vi "facade.vi"(0 "Data In":T13, 2 "Display State In":T3={"current frame index"=0, "number of images"=0, "ROI (frames)"={"ROI"=[]}, "control refs"={"frame"=refnum, "image"=refnum, "saveROIsButton"=refnum, "loadImageSwitch"=refnum, "loadROIsSwitch"=refnum, "saveROIsSwitch"=refnum, "loadImagePath"=refnum, "loadROIPath"=refnum, "redraw"=refnum}, "calibration"={"x"=0.0, "y"=0.0, "x unit"=enum."um", "y unit"=enum."um"}, "xpaths"={"x offset"="", "y offset"="", "z offset"=""}, "offset"=refnum, "XML description"="", "number of ROIs"=0.0, "ROI Tool Buttons Visible"={"Zoom Tool"=FALSE, "Selection Tool"=FALSE, "Pan Tool"=FALSE, "Point Tool"=FALSE, "Line Tool"=FALSE, "Rectangle Tool"=FALSE, "Rotated Rectangle Tool"=FALSE, "Polyline Tool"=FALSE, "Polygon Tool"=FALSE, "Freehand Tool"=FALSE, "Closed Freehand Tool"=FALSE, "Ellipse Tool"=FALSE, "Annulus Tool"=FALSE}, "ROI color"=0, "enable ROI numbering?"=FALSE, "selected path to save ROIs"=path "", "starting path"=path "", "loaded image path"=path "", "array of overlays"=[], "pointCollection"=refnum, "ROImode"=enum."IMAQROIs", "selected point ID"=0.0, "point radius"=0, "point colours"=[], "PlotAreaSize"={"Width"=0, "Height"=0}, "last action"=enum."not specified"} {"array of overlays"."overlay size" min=1}, 3 "Container State":T12, 5 "error in (no error)":errorcluster) -> (4 "error out":errorcluster, 6 "Data Out":T13, 7 "Display State Out":T3={"current frame index"=0, "number of images"=0, "ROI (frames)"={"ROI"=[]}, "control refs"={"frame"=refnum, "image"=refnum, "saveROIsButton"=refnum, "loadImageSwitch"=refnum, "loadROIsSwitch"=refnum, "saveROIsSwitch"=refnum, "loadImagePath"=refnum, "loadROIPath"=refnum, "redraw"=refnum}, "calibration"={"x"=0.0, "y"=0.0, "x unit"=enum."um", "y unit"=enum."um"}, "xpaths"={"x offset"="", "y offset"="", "z offset"=""}, "offset"=refnum, "XML description"="", "number of ROIs"=0.0, "ROI Tool Buttons Visible"={"Zoom Tool"=FALSE, "Selection Tool"=FALSE, "Pan Tool"=FALSE, "Point Tool"=FALSE, "Line Tool"=FALSE, "Rectangle Tool"=FALSE, "Rotated Rectangle Tool"=FALSE, "Polyline Tool"=FALSE, "Polygon Tool"=FALSE, "Freehand Tool"=FALSE, "Closed Freehand Tool"=FALSE, "Ellipse Tool"=FALSE, "Annulus Tool"=FALSE}, "ROI color"=0, "enable ROI numbering?"=FALSE, "selected path to save ROIs"=path "", "starting path"=path "", "loaded image path"=path "", "array of overlays"=[], "pointCollection"=refnum, "ROImode"=enum."IMAQROIs", "selected point ID"=0.0, "point radius"=0, "point colours"=[], "PlotAreaSize"={"Width"=0, "Height"=0}, "last action"=enum."not specified"} {"array of overlays"."overlay size" min=1}, 8 "Action":T2)   [LabVIEW 2010, in "XImage.xctl"]
uses:
  XImage.xctl
  data.ctl
  classes/ImageCollection/ImageCollection/ImageCollection.lvclass
  <vilib>/_xctls/Container State.ctl
  state.ctl
  classes/SpaceVector/SpaceVector/SpaceVector.lvclass
  classes/PointCollection/PointCollection/PointCollection.lvclass
  ROI_frames_cluster.ctl
  control_refs_cluster.ctl
  calibration_cluster.ctl
  enumerations/unit.ctl
  xpath_cluster.ctl
  overlays_cluster.ctl
  ROI_mode_enum.ctl
  last_action_enum.ctl
  <vilib>/_xctls/Action.ctl
  classes/Image/Image/Image.lvclass
  <vilib>/vision/Image Controls.llb/IMAQ Image.ctl
  <vilib>/Utility/inputDevices.llb/keyboardAcquire.vi
  <vilib>/Utility/inputDevices.llb/closeKeyboard.vi
  <vilib>/_xctls/XControlSupport.lvlib
panel:
  in  "button:saveLinear":bool
  out "event case no.":i32
  in  "redraw":bool
  in  "button:savePoints":bool
  in  "button:loadPoints":bool
  in  "showHeaderButton":bool
  in  "loadROIPath":path caption="start path"
  in  "loadImagePath":path
  in  "loadROIsSwitch":bool=TRUE
  in  "saveROIsSwitch":bool=TRUE
  in  "loadImageSwitch":bool=TRUE
  out "progress bar":u8(slide) scale=0.0..100.0
  in  "button:loadROIs":bool
  in  "button:saveROIs":bool
  in  "button:loadImage":bool
  in  "frame":i32(slide) scale=0.0..10.0
  out "Image":T1(plugin-control)
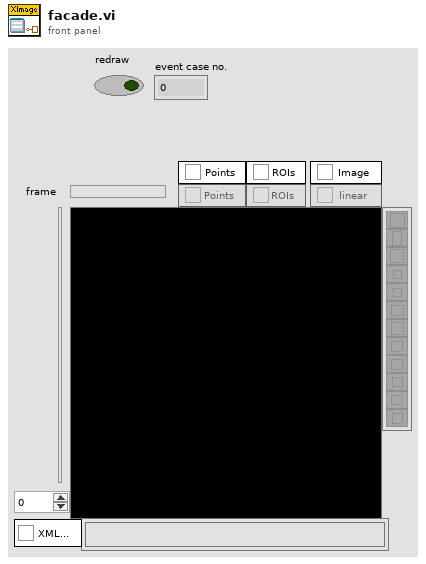
[diagram p1: front panel]
types:
  T1 = typedef "IMAQ Image.ctl" = refnum<image>
  T2 = typedef "XControlSupport.lvlib/Action.ctl" = cluster{"Data Changed?":bool, "State Changed?":bool, "Action Name":string}
  T3 = typedef "XImage.xctl/state.ctl" = cluster{"current frame index":i32, "number of images":i32, "ROI (frames)":T4, "control refs":T5, "calibration":T6, "xpaths":T8, "offset":refnum<class "SpaceVector.lvclass">, "XML description":string, "number of ROIs":dbl, "ROI Tool Buttons Visible":cluster{"Zoom Tool":bool, "Selection Tool":bool, "Pan Tool":bool, "Point Tool":bool, "Line Tool":bool, "Rectangle Tool":bool, "Rotated Rectangle Tool":bool, "Polyline Tool":bool, "Polygon Tool":bool, "Freehand Tool":bool, "Closed Freehand Tool":bool, "Ellipse Tool":bool, "Annulus Tool":bool}, "ROI color":u32, "enable ROI numbering?":bool, "selected path to save ROIs":path, "starting path":path, "loaded image path":path, "array of overlays":T9[], "pointCollection":refnum<class "PointCollection.lvclass">, "ROImode":T10, "selected point ID":dbl, "point radius":i32, "point colours":u32[], "PlotAreaSize":cluster{"Width":u32, "Height":u32}, "last action":T11}
  T4 = typedef "XImage.xctl/ROI_frames_cluster.ctl" = cluster{"ROI":cluster{"Global Rectangle":i32[], "Contours":cluster{"Contour Type":u32, "ROI Type":u32, "Points":i32[]}[]}[]}
  T5 = typedef "XImage.xctl/control_refs_cluster.ctl" = cluster{"frame":refnum<vi>, "image":refnum<vi>, "saveROIsButton":refnum<vi>, "loadImageSwitch":refnum<vi>, "loadROIsSwitch":refnum<vi>, "saveROIsSwitch":refnum<vi>, "loadImagePath":refnum<vi>, "loadROIPath":refnum<vi>, "redraw":refnum<vi>}
  T6 = typedef "XImage.xctl/calibration_cluster.ctl" = cluster{"x":dbl, "y":dbl, "x unit":T7, "y unit":T7}
  T7 = typedef "Image.lvclass/unit.ctl" = enum16{"um", "s"}
  T8 = typedef "XImage.xctl/xpath_cluster.ctl" = cluster{"x offset":string, "y offset":string, "z offset":string}
  T9 = typedef "XImage.xctl/overlays_cluster.ctl" = cluster{"overlay array":cluster{i32[][]}[], "overlay name":string, "color (red)":u32, "overlay size":i32, "overlay type":enum16{"crosshair", "circle"}}
  T10 = typedef "XImage.xctl/ROI_mode_enum.ctl" = enum16{"none", "IMAQROIs", "PointCollection"}
  T11 = typedef "XImage.xctl/last_action_enum.ctl" = enum16{"not specified", "image loaded", "frame changed", "ROIs changed"}
  T12 = typedef "XControlSupport.lvlib/Container State.ctl" = cluster{"Indicator?":bool, "Run Mode?":bool, " Refnum":refnum<vi>}
  T13 = typedef "XImage.xctl/data.ctl" = refnum<class "ImageCollection.lvclass">
  T14 = enum16{"0", "1", "2", "3", "4", "5", "6", "7", "8", "9", "A", "B", "C", "D", "E", "F", "G", "H", "I", "J", "K", "L", "M", "N", "O", "P", "Q", "R", "S", "T", "U", "V", "W", "X", "Y", "Z", "F1", "F2", "F3", "F4", "F5", "F6", "F7", "F8", "F9", "F10", "F11", "F12", "F13", "F14", "F15", "ADD", "BACK", "BACKSLASH", "CAPITAL", "COMMA", "DECIMAL", "DELETE", "DIVIDE", "DOWN", "END", "EQUALS", "ESCAPE", "GRAVE (`)", "HOME", "INSERT", "LBRACKET", "LCONTROL", "LEFT", "L ALT", "LSHIFT", "LWIN", "MINUS", "MULTIPLY", "NEXT", "NUMLOCK", "NUMPAD_0", "NUMPAD_1", "NUMPAD_2", "NUMPAD_3", "NUMPAD_4", "NUMPAD_5", "NUMPAD_6", "NUMPAD_7", "NUMPAD_8", "NUMPAD_9", "PAUSE", "PERIOD", "PRIOR (PG UP)", "RBRACKET", "RCONTROL", "RETURN", "RIGHT", "R ALT", "RSHIFT", "RWIN", "SCROLL", "SEMICOLON", "SLASH", "SPACE", "SUBTRACT", "TAB", "UP", "ENTER (num pad)", "' (quote)"}
  T15 = cluster{"Zoom Tool":bool, "Selection Tool":bool, "Pan Tool":bool, "Point Tool":bool, "Line Tool":bool, "Rectangle Tool":bool, "Rotated Rectangle Tool":bool, "Polyline Tool":bool, "Polygon Tool":bool, "Freehand Tool":bool, "Closed Freehand Tool":bool, "Ellipse Tool":bool, "Annulus Tool":bool}
  T16 = cluster{"Global Rectangle":i32[], "Contours":cluster{"Contour Type":u32, "ROI Type":u32, "Points":i32[]}[]}
  T17 = cluster{"Global Rectangle":i32[], "Contours":cluster{"Contour Type":u32, "ROI Type":u32, "Points":i32[]}[]}[]
  T18 = cluster{"Contour Type":u32, "ROI Type":u32, "Points":i32[]}[]
  T19 = enum8{"Enabled", "Disabled", "Disabled and Grayed Out"}
  T20 = typedef "Image Type" = u32
  T21 = enum16{"0", "1", "2", "3", "4", "5", "6", "7", "8", "9", "A", "B", "C", "D", "E", "F", "G", "H", "I", "J", "K", "L", "M", "N", "O", "P", "Q", "R", "S", "T", "U", "V", "W", "X", "Y", "Z", "F1", "F2", "F3", "F4", "F5", "F6", "F7", "F8", "F9", "F10", "F11", "F12", "F13", "F14", "F15", "ADD", "BACK", "BACKSLASH", "CAPITAL", "COMMA", "DECIMAL", "DELETE", "DIVIDE", "DOWN", "END", "EQUALS", "ESCAPE", "GRAVE (`)", "HOME", "INSERT", "LBRACKET", "LCONTROL", "LEFT", "L ALT", "LSHIFT", "LWIN", "MINUS", "MULTIPLY", "NEXT", "NUMLOCK", "NUMPAD_0", "NUMPAD_1", "NUMPAD_2", "NUMPAD_3", "NUMPAD_4", "NUMPAD_5", "NUMPAD_6", "NUMPAD_7", "NUMPAD_8", "NUMPAD_9", "PAUSE", "PERIOD", "PRIOR (PG UP)", "RBRACKET", "RCONTROL", "RETURN", "RIGHT", "R ALT", "RSHIFT", "RWIN", "SCROLL", "SEMICOLON", "SLASH", "SPACE", "SUBTRACT", "TAB", "UP", "ENTER (num pad)", "' (quote)"}[]
  T22 = typedef "LVRectTypeDef.ctl" = cluster{"left":i16, "top":i16, "right":i16, "bottom":i16}
  T23 = typedef "LVBoundsTypeDef.ctl" = cluster{"Width":u32, "Height":u32}
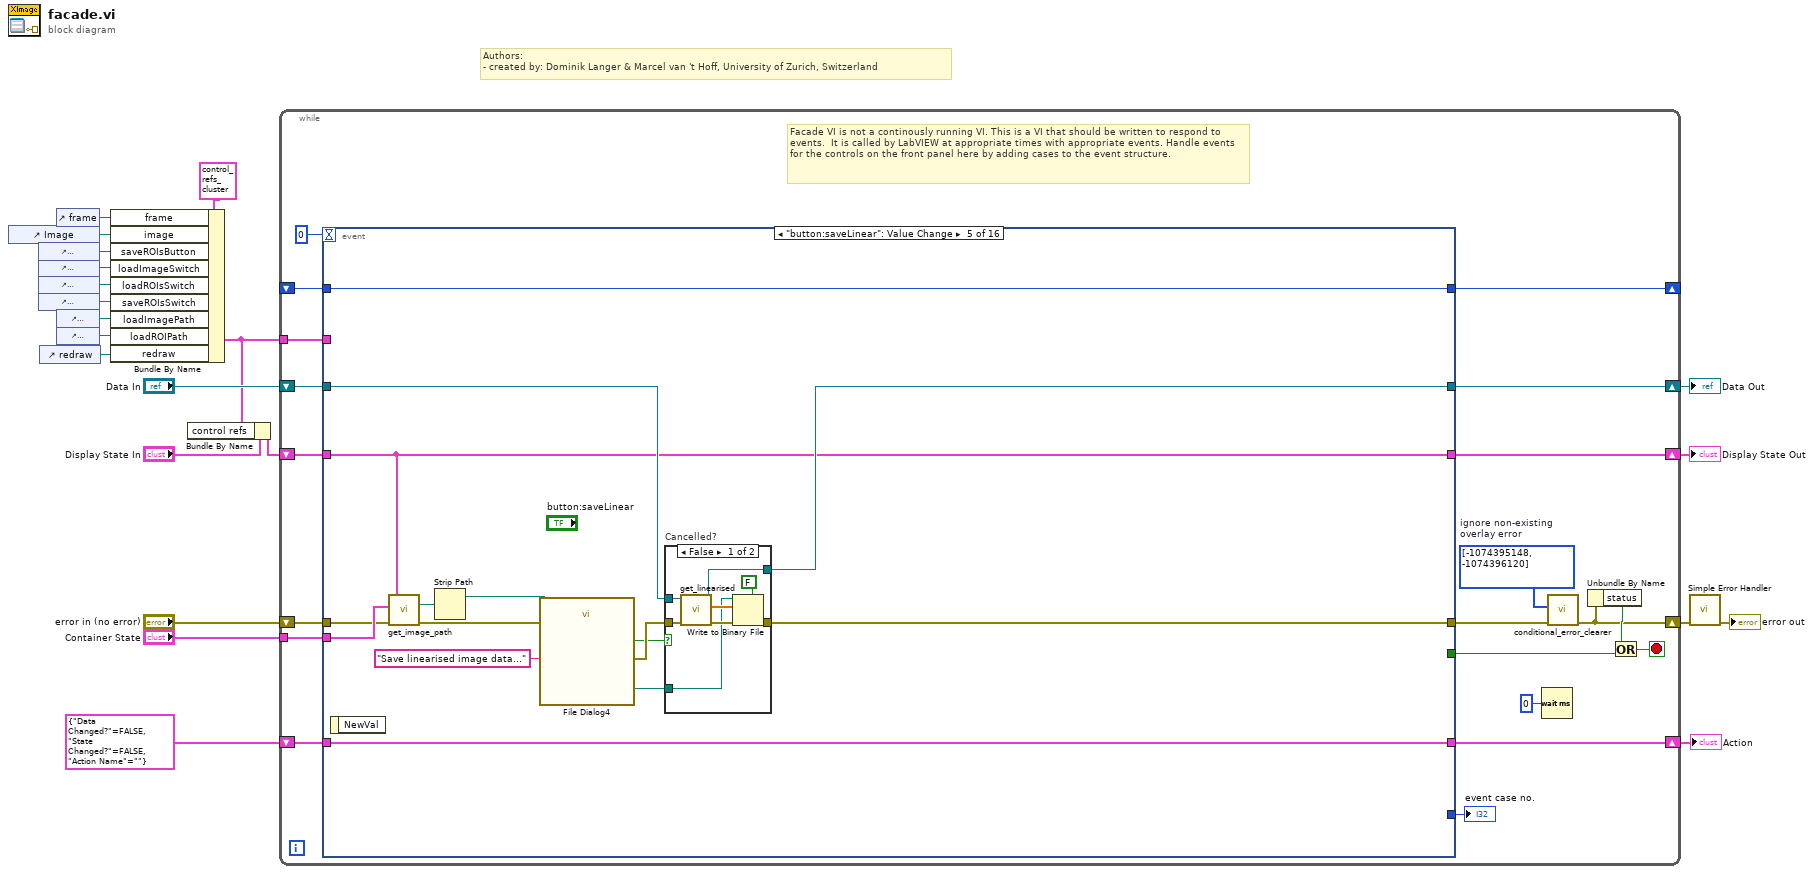
[diagram p0: block diagram]
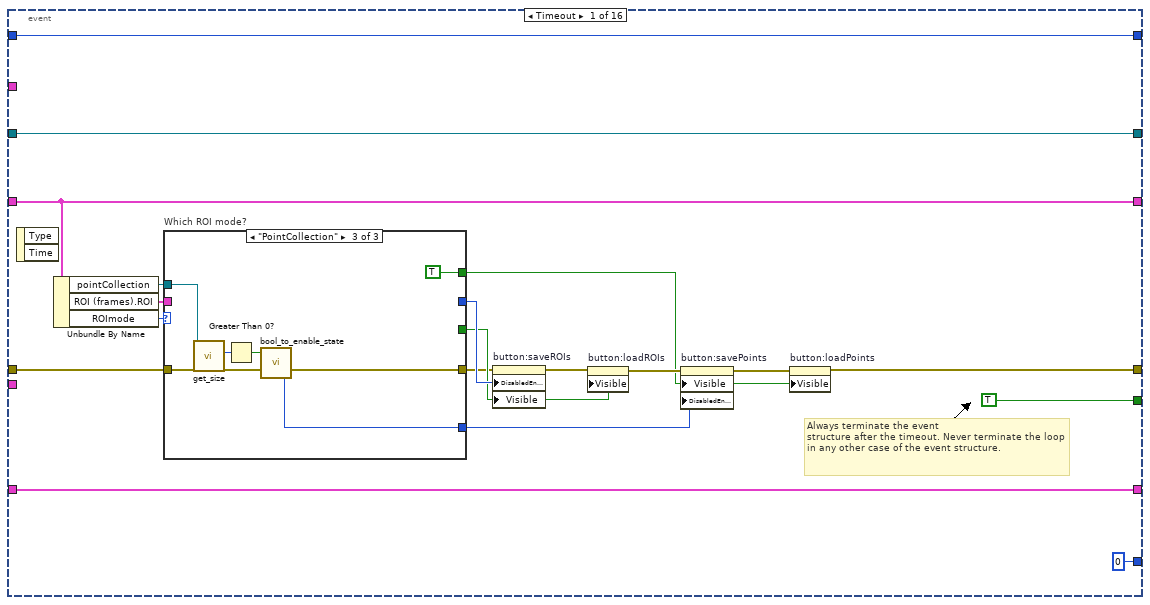
[diagram p2: hidden frame]
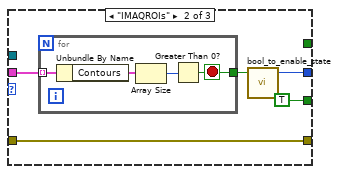
[diagram p4: hidden frame]
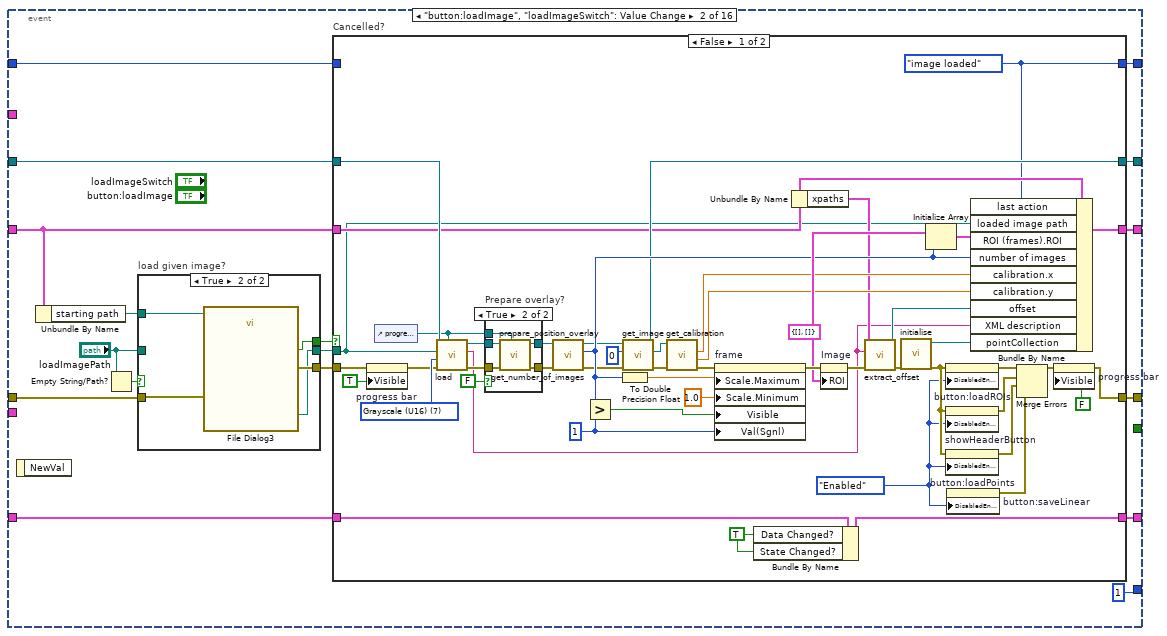
[diagram p5: hidden frame]
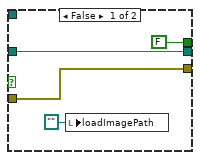
[diagram p6: hidden frame]
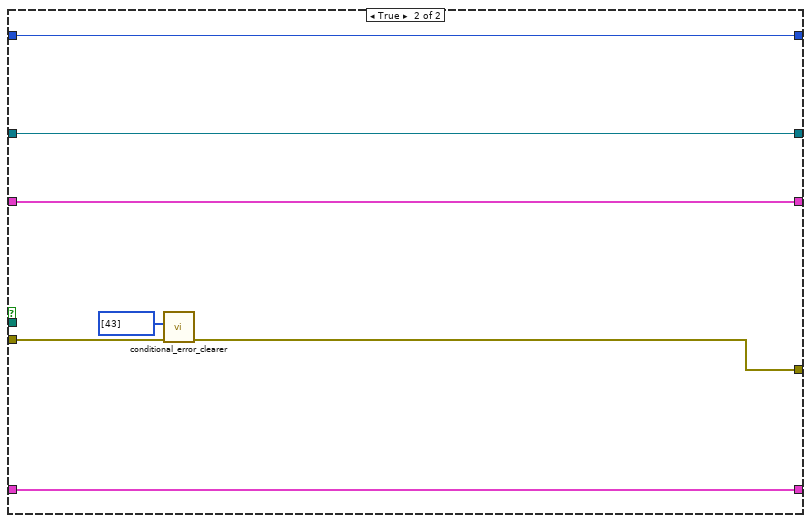
[diagram p8: hidden frame]
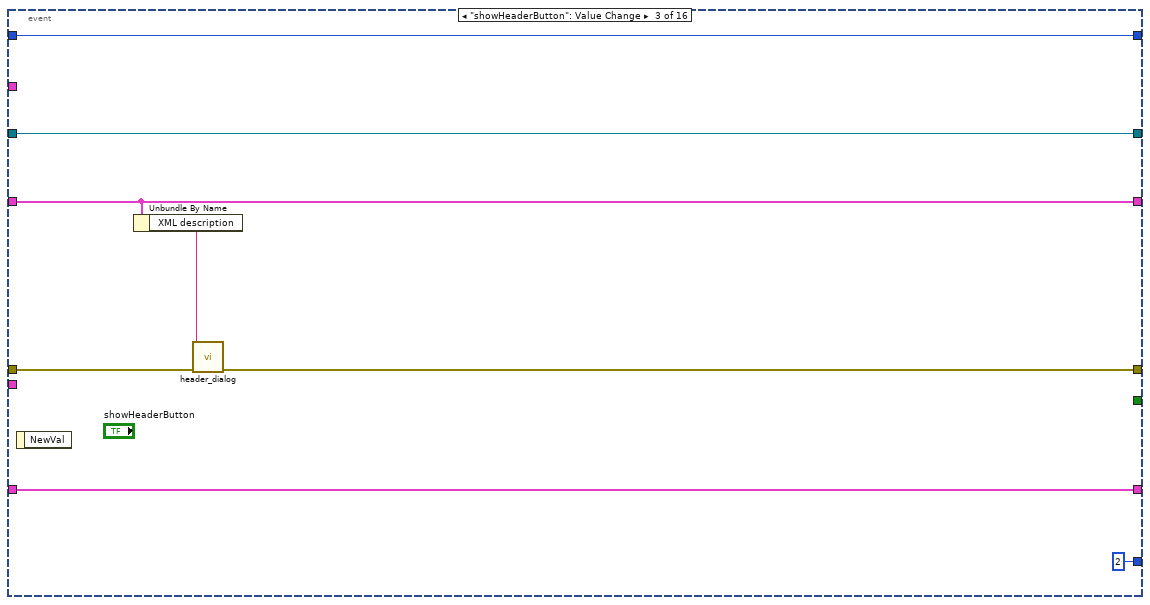
[diagram p9: hidden frame]
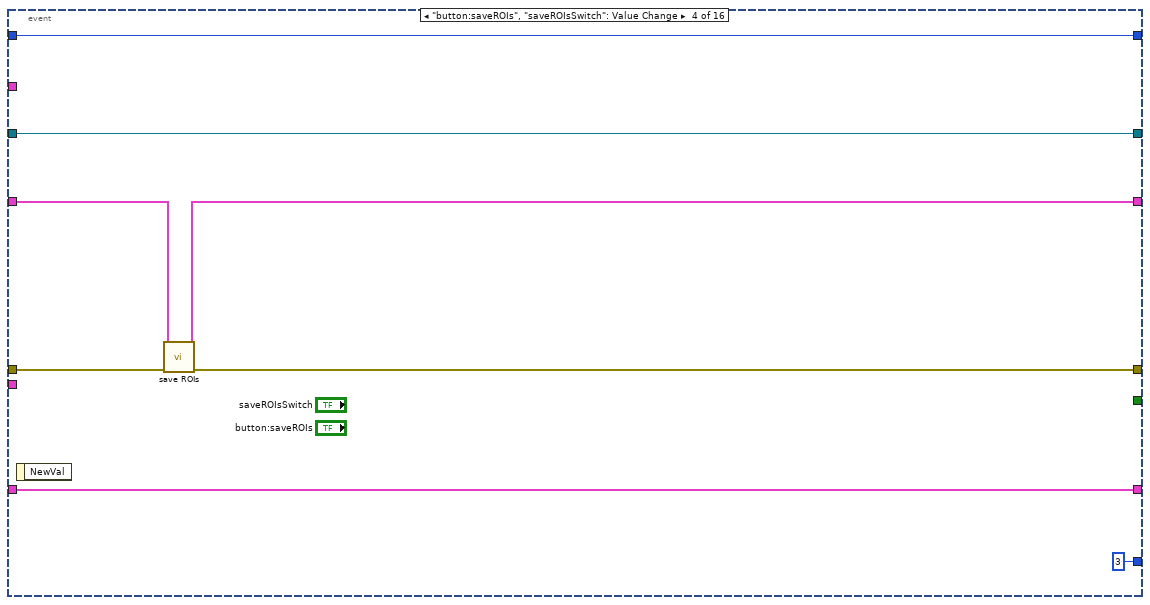
[diagram p10: hidden frame]
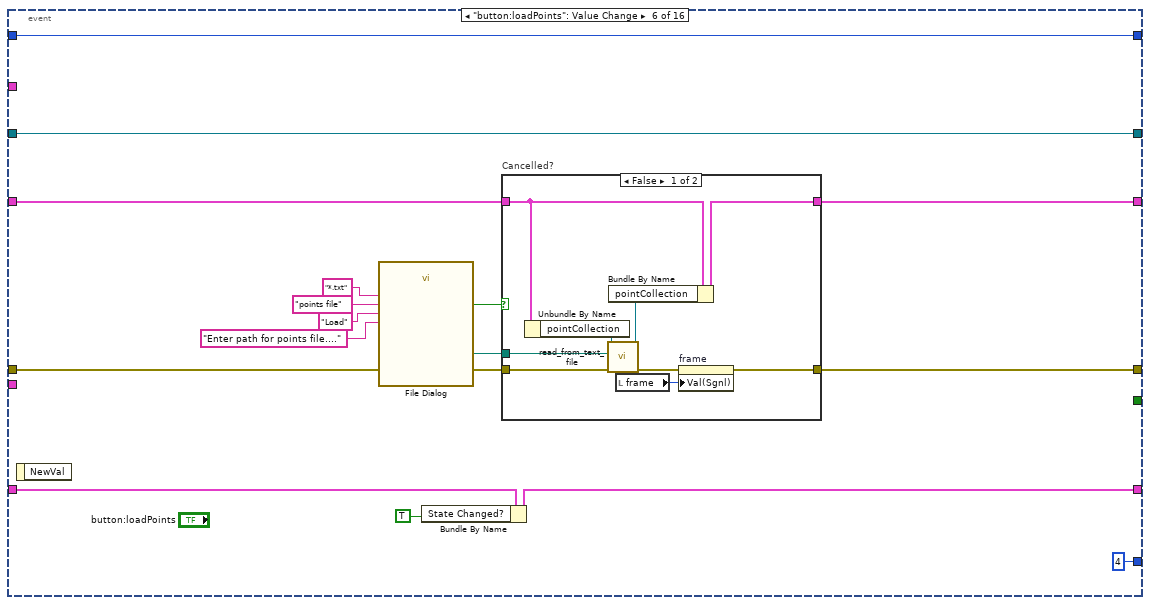
[diagram p12: hidden frame]
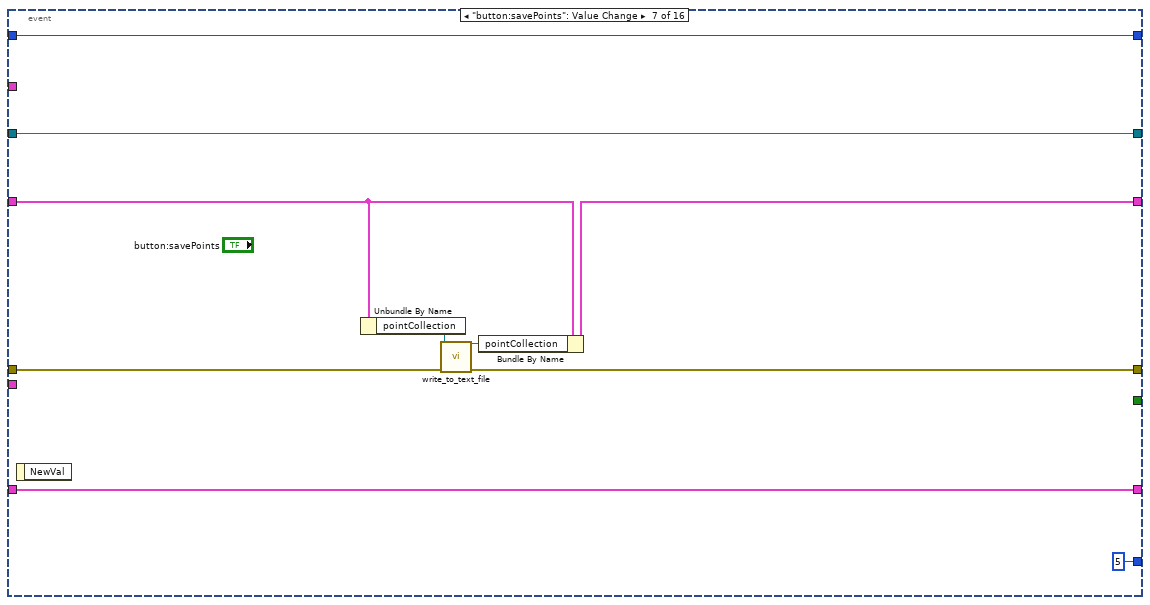
[diagram p14: hidden frame]
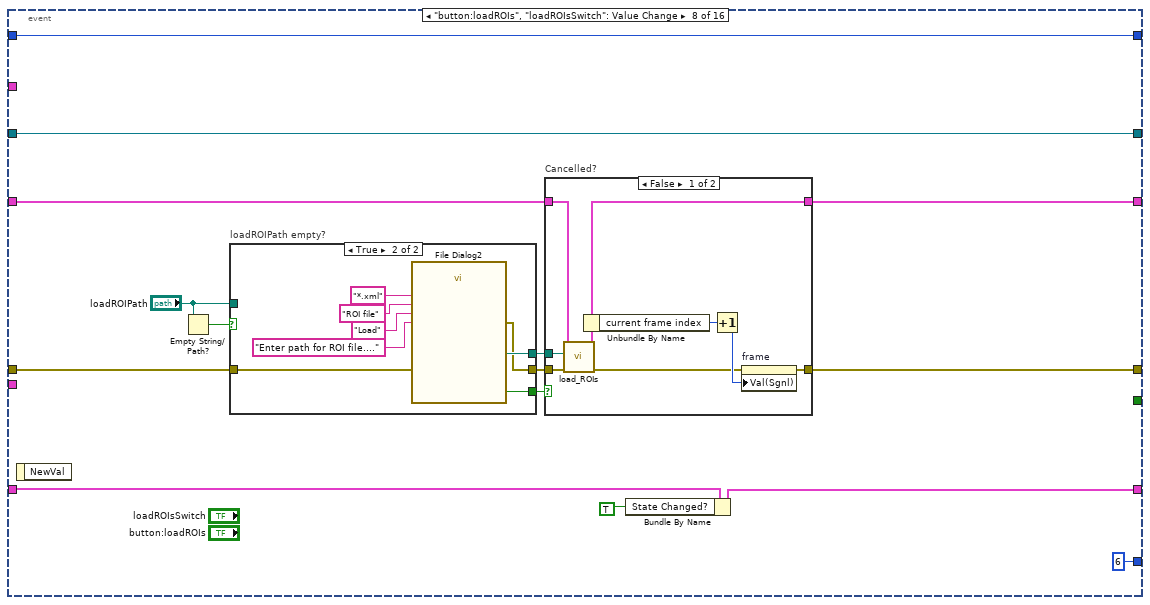
[diagram p15: hidden frame]
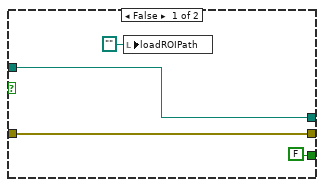
[diagram p16: hidden frame]
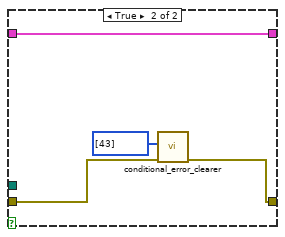
[diagram p17: hidden frame]
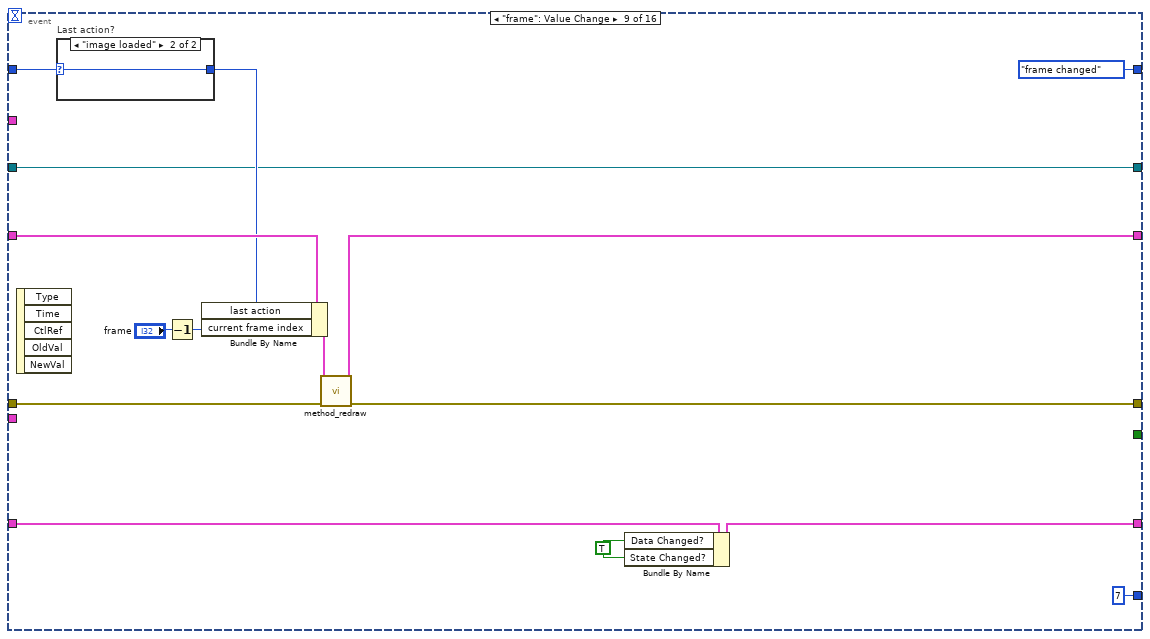
[diagram p18: hidden frame]
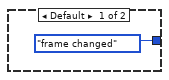
[diagram p19: hidden frame]
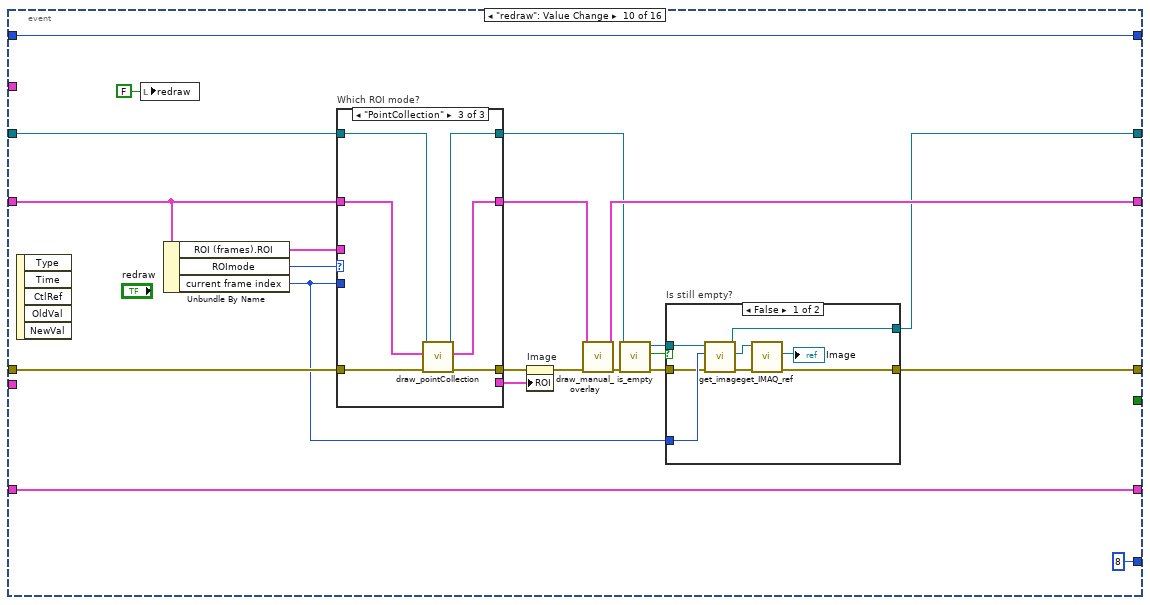
[diagram p20: hidden frame]
diagram:
  # "Authors: \n- created by: Dominik Langer & Marcel van 't Hoff, University of Zurich, Switzerland"
  n1 = control-ref of="Image"() -> (w8:refnum<vi>)
  n2 = control-ref of="button:saveROIs"() -> (w9:refnum<vi>)
  n3 = control-ref of="loadImageSwitch"() -> (w10:refnum<vi>)
  n4 = control-ref of="loadROIsSwitch"() -> (w11:refnum<vi>)
  n5 = control-ref of="saveROIsSwitch"() -> (w12:refnum<vi>)
  n6 = control-ref of="redraw"() -> (w6:refnum<vi>)
  n7 = control-ref of="frame"() -> (w7:refnum<vi>)
  n8 = control-ref of="loadImagePath"() -> (w13:refnum<vi>)
  n9 = control-ref of="loadROIPath"() -> (w5:refnum<vi>)
  n10 = Bundle By Name(cluster=T5 {"frame"=refnum, "image"=refnum, "saveROIsButton"=refnum, "loadImageSwitch"=refnum, "loadROIsSwitch"=refnum, "saveROIsSwitch"=refnum, "loadImagePath"=refnum, "loadROIPath"=refnum, "redraw"=refnum} ("control refs"), "frame"=w7, "image"=w8, "saveROIsButton"=w9, "loadImageSwitch"=w10, "loadROIsSwitch"=w11, "saveROIsSwitch"=w12, "loadImagePath"=w13, "loadROIPath"=w5, "redraw"=w6) -> (w1:T5)
  n11 = Bundle By Name(cluster="Display State In", "control refs"=w1) -> (w2:T3)
  n12 = while {
    shift-right: [w42] -> w19
    shift-left: w2 -> [w26]
    tunnel: "Container State" -> [w40]
    shift-right: [w38] -> w22
    shift-left: "Data In" -> [w39]
    shift-right: [w32] -> w18
    shift-left: T2 {"Data Changed?"=FALSE, "State Changed?"=FALSE, "Action Name"=""} ("Action") -> [w37]
    shift-right: [w31] -> w15
    shift-left: "error in (no error)" -> [w36]
    shift-right: [w28] -> _
    shift-left: _ -> [w27]
    tunnel: w1 -> [w23]
    stop <- w34 stop-if-true
    w29 = i32[] [-1074395148, -1074396120]  # ignore non-existing overlay error
    # "Facade VI is not a continously running VI. This is a VI that should be written to respond to events.  It is called by LabVIEW at appropriate times with appropriate events. Handle events for the controls on the front panel here by adding cases to the event structure."
    n13 = event shown="[4] \"button:saveLinear\": Value Change" {
      selector: _ -> [_ _ _ _ _ _ _ _ _ _ _ _ _ _ _ _]
      dyn-events: _ -> [_ _ _ _ _ _ _ _ _ _ _ _ _ _ _ _]
      timeout: 0 -> [_ _ _ _ _ _ _ _ _ _ _ _ _ _ _ _]
      tunnel: w26 -> [w58 w83 w174 w179 w190 w224 w241 w256 w297 w318 w365 w495 w505 w538 w555 _]
      tunnel: [w58 w92 w174 w182 w190 w223 w240 w260 w289 w314 w354 w494 w503 w538 w554 w639] -> w42
      tunnel: [TRUE _ _ _ _ _ _ _ _ _ _ _ _ _ _ _] -> w35
      tunnel: w40 -> [_ _ _ _ w189 _ _ _ _ _ _ _ w523 w539 w559 w640]
      tunnel: w39 -> [w60 w93 w176 w184 w197 w225 w243 w261 w287 w312 w358 w497 w507 w537 w607 w614]
      tunnel: [w60 w91 w176 w184 w194 w225 w243 w261 w287 w308 w359 w496 w507 w537 w607 T13 refnum ("imageCollection")] -> w38
      tunnel: [w59 w94 w175 w183 w199 w220 w246 w258 w298 w324 w361 w492 w524 w536 w550 w636] -> w32
      tunnel: w37 -> [w59 w95 w175 w183 w199 w221 w246 w259 w299 w324 w362 w493 w524 w536 w551 w637]
      tunnel: w36 -> [w46 w87 w172 w180 w188 w214 w245 w252 w286 w311 w363 w491 w521 w533 w558 w613]
      tunnel: [w48 w86 w171 w181 w196 w219 w244 w251 w288 w309 w356 w490 w504 w532 w574 w609] -> w30
      tunnel: [w56 w81 w170 w178 w198 w211 w238 w248 last_action_enum."frame changed" ("last action") w323 w360 w480 w509 w531 w549 w621] -> w28
      tunnel: w27 -> [w56 w80 w170 w178 w198 w211 w238 w248 w294 w323 w360 w480 w509 w531 w549 w621]
      tunnel: [0 1 2 3 _ 4 5 6 7 8 9 10 11 12 13 14] -> w25
      tunnel: w23 -> [_ _ _ _ _ _ _ _ _ _ _ _ _ _ _ w618]
      event Timeout {
        # "Always terminate the event\nstructure after the timeout. Never terminate the loop in any other case of the event structure."
        n14 = event-data() -> ()  [unwired: 1 in, 2 out]
        n15 = Unbundle By Name(w58) -> ("pointCollection"=w47:refnum<class "PointCollection.lvclass">, "ROI (frames).ROI"=w57:T17, "ROImode"=w55:T10)
        n16 = case "Which ROI mode?" shown="\"PointCollection\"" w55 {
          tunnel: w57 -> [_ w67 _]
          tunnel: [_ w65 _] -> w54
          tunnel: [_ TRUE _] -> w52
          tunnel: [_ _ TRUE] -> w49
          tunnel: w47 -> [_ _ w76]
          tunnel: w46 -> [w62 w63 w77]
          tunnel: [w62 w63 w75] -> w45
          tunnel: [_ _ w72] -> w44
          frame "none", Default {
          }
          frame "IMAQROIs" {
            n17 = for {
              tunnel: w67 -> [w71] mode=indexing
              tunnel: [w68] -> w66
              stop <- w68 stop-if-true
              n18 = Unbundle By Name(w71) -> ("Contours"=w70:T18)
              n19 = Array Size(array=w70) -> (size(s)=w69:i32)
              n20 = Greater Than 0?(x=w69) -> (x > 0?=w68:bool)
            }
            n21 = call "bool_to_enable_state.vi"("boolean in"=w66) -> ("enabled status out"=w65:T19)  [unwired: 4 in]
          }
          frame "PointCollection" {
            n22 = call "get_size.vi"("error in (no error)"=w77, "PointCollection in"=w76) -> ("error out"=w75:errorcluster, "number of points"=w74:i32)  [unwired: 7 in, 1 out]
            n23 = Greater Than 0?(x=w74) -> (x > 0?=w73:bool)
            n24 = call "bool_to_enable_state.vi"("boolean in"=w73) -> ("enabled status out"=w72:T19)  [unwired: 4 in]
          }
        }
        n25 = property on="button:saveROIs" class="Bool"(error in=w45, "DisabledEnum"=w54, "Visible"=w52) -> (error out=w53:errorcluster)  [unwired: 1 in, 1 out]
        n26 = property on="button:loadROIs" class="Bool"(error in=w53, "Visible"=w52) -> (error out=w51:errorcluster)  [unwired: 1 in, 1 out]
        n27 = property on="button:savePoints" class="Bool"(error in=w51, "Visible"=w49, "DisabledEnum"=w44) -> (error out=w50:errorcluster)  [unwired: 1 in, 1 out]
        n28 = property on="button:loadPoints" class="Bool"(error in=w50, "Visible"=w49) -> (error out=w48:errorcluster)  [unwired: 1 in, 1 out]
      }
      event "button:loadImage", "loadImageSwitch": Value Change {
        n29 = event-data() -> ()  [unwired: 1 in, 1 out]
        n30 = Unbundle By Name(w83) -> ("starting path"=w82:path)
        n31 = Empty String/Path?(string/path="loadImagePath") -> (empty?=w85:bool)
        n32 = case "load given image?" shown="True" w85 {
          tunnel: [w98 w104] -> w90
          tunnel: [w99 w103] -> w89
          tunnel: [FALSE ("cancelled") w102] -> w88
          tunnel: w87 -> [w98 w101]
          tunnel: "loadImagePath" -> [w99 _]
          tunnel: w82 -> [_ w100]
          frame False {
            n33 = local write "loadImagePath"(path "") -> ()
          }
          frame True {
            n34 = call "File Dialog3"("start path"=w100, "error in"=w101) -> ("selected path"=w103:path, "cancelled"=w102:bool, "error out"=w104:errorcluster)  [unwired: 10 in, 1 out]
          }
        }
        n35 = case "Cancelled?" shown="False" w88 {
          tunnel: w95 -> [w151 w166]
          tunnel: [w150 w166] -> w94
          tunnel: w93 -> [w148 w168]
          tunnel: w83 -> [w126 w167]
          tunnel: [w146 w167] -> w92
          tunnel: [w131 w168] -> w91
          tunnel: w90 -> [w140 w165]
          tunnel: w89 -> [w107 _]
          tunnel: [w124 w164] -> w86
          tunnel: [w108 w162] -> w81
          tunnel: w80 -> [_ w162]
          frame False {
            w108 = last_action_enum."image loaded" ("last action")
            w106 = T19."Enabled" ("Disabled")
            w143 = T16 {"Global Rectangle"=[], "Contours"=[]} ("ROI")
            w147 = T20 7 items=["Grayscale (U8)", "Grayscale (I16)", "Grayscale (SGL)", "Complex (CSG)", "RGB (U32)", "HSL (U32)", "RGB (U64)", "Grayscale (U16)"] ("Image Type")
            w109 = TRUE ("Data Changed?")
            w149 = 1 ("y")
            n36 = property on="progress bar" class="Slide (strict)"(error in=w140, "Visible"=TRUE) -> (error out=w139:errorcluster)  [unwired: 1 in, 1 out]
            n37 = control-ref of="progress bar"() -> (w119:refnum<vi>)
            n38 = call "load.vi"("progress bar ref"=w119, "error in (no error)"=w139, "Image Type"=w147, "path in"=w107, "ImageCollection in"=w148) -> ("error out"=w123:errorcluster, "description"=w118:string, "ImageCollection out"=w121:T13)  [unwired: 2 in, 2 out]
            n39 = case "Prepare overlay?" shown="True" FALSE {
              tunnel: w123 -> [w156 w161]
              tunnel: [w156 w160] -> w122
              tunnel: w121 -> [w155 w159]
              tunnel: [w155 w158] -> w120
              tunnel: w119 -> [_ w157]
              frame False {
              }
              frame True {
                n40 = call "prepare_position_overlay.vi"("progress bar ref"=w157, "error in (no error)"=w161, "ImageCollection in"=w159) -> ("error out"=w160:errorcluster, "ImageCollection out"=w158:T13)  [unwired: 6 in, 1 out]
              }
            }
            n41 = call-dynamic "get_number_of_images.vi"("error in (no error)"=w122, "ImageCollection in"=w120) -> ("error out"=w134:errorcluster, "size"=w142:i32, "ImageCollection out"=w132:T13)  [unwired: 7 in]
            n42 = Greater?(x=w142, y=w149) -> (0:w152:bool)
            n43 = To Double Precision Float(number=w142) -> (double precision float=w154:dbl)
            n44 = call-dynamic "get_image.vi"("error in (no error)"=w134, "index"=0, "ImageCollection in"=w132) -> ("error out"=w137:errorcluster, "Image.lvclass"=w136:refnum<class "Image.lvclass">, "ImageCollection out"=w131:T13)  [unwired: 6 in]
            n45 = call "get_calibration.vi"("error in (no error)"=w137, "Image.lvclass in"=w136) -> ("error out"=w133:errorcluster, "y"=w129:dbl, "x"=w130:dbl)  [unwired: 2 in, 5 out]
            n46 = property on="frame" class="Slide (strict)"(error in=w133, "Scale.Maximum"=w154, "Scale.Minimum"=1.0 ("Scale.Range:Minimum"), "Visible"=w152, "Val(Sgnl)"=w149) -> (error out=w144:errorcluster)  [unwired: 1 in, 1 out]
            n47 = Bundle By Name(cluster=w151, "Data Changed?"=w109, "State Changed?"=w109) -> (w150:T2)
            n48 = Unbundle By Name(w126) -> ("xpaths"=w125:T8)
            n49 = property on="Image" class="ImageControl"(error in=w144, "ROI"=w143) -> (error out=w128:errorcluster)  [unwired: 1 in, 1 out]
            n50 = call "extract_offset.vi"("error in (no error)"=w128, "xml header string"=w118, "xpaths"=w125) -> ("error out"=w112:errorcluster, "offset"=w127:refnum<class "SpaceVector.lvclass">)  [unwired: 7 in]
            n51 = call "initialise.vi"("error in (no error)"=w112) -> ("error out"=w111:errorcluster, "PointCollection out"=w110:refnum<class "PointCollection.lvclass">)  [unwired: 9 in]
            n52 = Initialize Array(w143, w142) -> (w145:T17)
            n53 = property on="button:loadROIs" class="Bool"(error in=w111, "DisabledEnum"=w106) -> (error out=w116:errorcluster)  [unwired: 1 in, 1 out]
            n54 = property on="showHeaderButton" class="Bool"(error in=w111, "DisabledEnum"=w106) -> (error out=w113:errorcluster)  [unwired: 1 in, 1 out]
            n55 = property on="button:loadPoints" class="Bool"(error in=w111, "DisabledEnum"=w106) -> (error out=w114:errorcluster)  [unwired: 1 in, 1 out]
            n56 = property on="button:saveLinear" class="Bool"("DisabledEnum"=w106) -> (error out=w105:errorcluster)  [unwired: 2 in, 1 out]
            n57 = Bundle By Name(cluster=w126, "last action"=w108, "loaded image path"=w107, "ROI (frames).ROI"=w145, "number of images"=w142, "calibration.x"=w130, "calibration.y"=w129, "offset"=w127, "XML description"=w118, "pointCollection"=w110) -> (w146:T3)
            n58 = Merge Errors(w116, w113, w114, w105) -> (w115:errorcluster)
            n59 = property on="progress bar" class="Slide (strict)"(error in=w115, "Visible"=FALSE) -> (error out=w124:errorcluster)  [unwired: 1 in, 1 out]
          }
          frame True {
            n60 = call "conditional_error_clearer.vi"("error in (no error)"=w165, "array of clearable error codes"=i32[] [43]) -> ("error out"=w164:errorcluster)  [unwired: 9 in]
          }
        }
      }
      event "showHeaderButton": Value Change {
        n61 = event-data() -> ()  [unwired: 1 in, 1 out]
        n62 = Unbundle By Name(w174) -> ("XML description"=w173:string)
        n63 = call "header_dialog.vi"("error in (no error)"=w172, "header string in"=w173) -> ("error out"=w171:errorcluster)  [unwired: 9 in]
      }
      event "button:saveROIs", "saveROIsSwitch": Value Change {
        n64 = event-data() -> ()  [unwired: 1 in, 1 out]
        n65 = call "save ROIs.vi"("error out"=w180, "Display State in"=w179) -> ("error out"=w181:errorcluster, "Display State out"=w182:T3)  [unwired: 7 in, 1 out]
      }
      event "button:saveLinear": Value Change {
        n66 = event-data() -> ()  [unwired: 1 in, 1 out]
        n67 = call "get_image_path.vi"("error in (no error)"=w188, "Container State"=w189, "Display State In"=w190) -> ("error out"=w187:errorcluster, "Value"=w186:path)  [unwired: 2 in, 1 out]
        n68 = Strip Path(path=w186) -> (stripped path=w185:path)  [unwired: 1 out]
        n69 = call "File Dialog4"("start path"=w185, "prompt"="Save linearised image data...", "error in"=w187) -> ("selected path"=w192:path, "cancelled"=w193:bool, "error out"=w195:errorcluster)  [unwired: 9 in, 1 out]
        n70 = case "Cancelled?" shown="False" w193 {
          tunnel: w197 -> [w207 w208]
          tunnel: [w204 w209] -> w196
          tunnel: w195 -> [w203 w209]
          tunnel: [w202 w208] -> w194
          tunnel: w192 -> [w201 _]
          frame False {
            n71 = call "get_linearised.vi"("error in (no error)"=w203, "ImageCollection in"=w207) -> ("error out"=w205:errorcluster, "pixels"=w206:sgl[], "ImageCollection out"=w202:T13)  [unwired: 7 in]
            n72 = Write to Binary File(file (use dialog)=w201, data=w206, error in=w205, 5:FALSE ("prepend array or string size? (T)")) -> (error out=w204:errorcluster)  [unwired: 2 in, 2 out]
          }
          frame True {
          }
        }
      }
      event "button:loadPoints": Value Change {
        n73 = event-data() -> ()  [unwired: 1 in, 1 out]
        n74 = call "File Dialog"("prompt"="Enter path for points file....", "button label"="Load", "error in"=w214, "pattern (all files)"="*.txt", "pattern label"="points file") -> ("selected path"=w213:path, "cancelled"=w212:bool)  [unwired: 7 in, 2 out]
        n75 = Bundle By Name(cluster=w221, "State Changed?"=TRUE) -> (w220:T2)
        n76 = case "Cancelled?" shown="False" w212 {
          tunnel: w224 -> [w232 w236]
          tunnel: [w231 w236] -> w223
          tunnel: [w229 w235] -> w219
          tunnel: w214 -> [w227 w235]
          tunnel: w213 -> [w226 _]
          frame False {
            n77 = Unbundle By Name(w232) -> ("pointCollection"=w233:refnum<class "PointCollection.lvclass">)
            n78 = call "read_from_text_file.vi"("error in (no error)"=w227, "file (use dialog)"=w226, "PointCollection in"=w233) -> ("error out"=w230:errorcluster, "PointCollection out"=w234:refnum<class "PointCollection.lvclass">)  [unwired: 7 in]
            n79 = Bundle By Name(cluster=w232, "pointCollection"=w234) -> (w231:T3)
            n80 = local read "frame"() -> (w228:i32)
            n81 = property on="frame" class="Slide (strict)"(error in=w230, "Val(Sgnl)"=w228) -> (error out=w229:errorcluster)  [unwired: 1 in, 1 out]
          }
          frame True {
          }
        }
      }
      event "button:savePoints": Value Change {
        n82 = event-data() -> ()  [unwired: 1 in, 1 out]
        n83 = Unbundle By Name(w241) -> ("pointCollection"=w242:refnum<class "PointCollection.lvclass">)
        n84 = call "write_to_text_file.vi"("error in (no error)"=w245, "PointCollection in"=w242) -> ("error out"=w244:errorcluster, "PointCollection out"=w239:refnum<class "PointCollection.lvclass">)  [unwired: 8 in]
        n85 = Bundle By Name(cluster=w241, "pointCollection"=w239) -> (w240:T3)
      }
      event "button:loadROIs", "loadROIsSwitch": Value Change {
        n86 = event-data() -> ()  [unwired: 1 in, 1 out]
        n87 = Empty String/Path?(string/path="loadROIPath") -> (empty?=w249:bool)
        n88 = case "loadROIPath empty?" shown="True" w249 {
          tunnel: [w263 w273] -> w255
          tunnel: [w265 w272] -> w254
          tunnel: [FALSE ("cancelled") w271] -> w253
          tunnel: w252 -> [w265 w266]
          tunnel: "loadROIPath" -> [w263 _]
          frame False {
            n89 = local write "loadROIPath"(path "") -> ()
          }
          frame True {
            n90 = call "File Dialog2"("prompt"="Enter path for ROI file....", "button label"="Load", "error in"=w266, "pattern (all files)"="*.xml", "pattern label"="ROI file") -> ("selected path"=w273:path, "cancelled"=w271:bool, "error out"=w272:errorcluster)  [unwired: 7 in, 1 out]
          }
        }
        n91 = case "Cancelled?" shown="False" w253 {
          tunnel: [w274 w285] -> w260
          tunnel: w256 -> [w276 w285]
          tunnel: w255 -> [w278 _]
          tunnel: w254 -> [w277 w283]
          tunnel: [w279 w282] -> w251
          frame False {
            n92 = call "load_ROIs.vi"("error in"=w277, "selected path"=w278, "Display State in"=w276) -> ("error out"=w275:errorcluster, "Display State out"=w274:T3)  [unwired: 7 in]
            n93 = Unbundle By Name(w274) -> ("current frame index"=w281:i32)
            n94 = Increment(x=w281) -> (x+1=w280:i32)
            n95 = property on="frame" class="Slide (strict)"(error in=w275, "Val(Sgnl)"=w280) -> (error out=w279:errorcluster)  [unwired: 1 in, 1 out]
          }
          frame True {
            n96 = call "conditional_error_clearer.vi"("error in (no error)"=w283, "array of clearable error codes"=i32[] [43]) -> ("error out"=w282:errorcluster)  [unwired: 9 in]
          }
        }
        n97 = Bundle By Name(cluster=w259, "State Changed?"=TRUE) -> (w258:T2)
      }
      event "frame": Value Change {
        w296 = TRUE ("State Changed?")
        n98 = event-data() -> ()  [unwired: 1 in, 5 out]
        n99 = case "Last action?" shown="\"image loaded\"" w294 {
          selector: w294 -> [_ w302]
          tunnel: [last_action_enum."frame changed" ("last action") w302] -> w293
          frame Default {
          }
          frame "image loaded" {
          }
        }
        n100 = Decrement(x="frame") -> (x-1=w295:i32)
        n101 = Bundle By Name(cluster=w297, "last action"=w293, "current frame index"=w295) -> (w290:T3)
        n102 = call "method_redraw.vi"("Display State In"=w290, "error in (no error)"=w286) -> ("Display State Out"=w289:T3, "error out"=w288:errorcluster)  [unwired: 12 in]
        n103 = Bundle By Name(cluster=w299, "Data Changed?"=w296, "State Changed?"=w296) -> (w298:T2)
      }
      event "redraw": Value Change {
        n104 = event-data() -> ()  [unwired: 1 in, 5 out]
        n105 = local write "redraw"(FALSE ("redraw")) -> ()
        n106 = Unbundle By Name(w318) -> ("ROI (frames).ROI"=w313:T17, "ROImode"=w319:T10, "current frame index"=w310:i32)
        n107 = case "Which ROI mode?" shown="\"PointCollection\"" w319 {
          tunnel: w318 -> [w336 w341 w346]
          tunnel: [w336 w340 w351] -> w315
          tunnel: w311 -> [w337 w343 w349]
          tunnel: [w337 w342 w348] -> w320
          tunnel: [w335 w344 w350] -> w303
          tunnel: [_ w345 _] -> w321
          tunnel: w312 -> [w335 w344 w347]
          tunnel: w310 -> [_ w339 _]
          tunnel: w313 -> [_ w338 _]
          frame "none", Default {
          }
          frame "IMAQROIs" {
            n108 = Index Array(array=w338, index=w339) -> (element=w345:T16)
            n109 = call "number_ROIs.vi"("error in"=w343, "Display State In"=w341) -> ("error out"=w342:errorcluster, "Display State Out"=w340:T3)  [unwired: 8 in]
          }
          frame "PointCollection" {
            n110 = call "draw_pointCollection.vi"("error in (no error)"=w349, "Display State In"=w346, "ImageCollection in"=w347) -> ("error out"=w348:errorcluster, "Display State Out"=w351:T3, "ImageCollection out"=w350:T13)  [unwired: 6 in]
          }
        }
        n111 = property on="Image" class="ImageControl"(error in=w320, "ROI"=w321) -> (error out=w316:errorcluster)  [unwired: 1 in, 1 out]
        n112 = call "draw_manual_overlay.vi"("error in"=w316, "Display State In"=w315) -> ("error out"=w307:errorcluster, "Display State Out"=w314:T3)  [unwired: 8 in]
        n113 = call "is_empty.vi"("error in (no error)"=w307, "ImageCollection in"=w303) -> ("error out"=w306:errorcluster, "is empty?"=w304:bool, "ImageCollection out"=w305:T13)  [unwired: 7 in]
        n114 = case "Is still empty?" shown="False" w304 {
          tunnel: w310 -> [w329 _]
          tunnel: [w328 w334] -> w309
          tunnel: [w327 w333] -> w308
          tunnel: w306 -> [w326 w334]
          tunnel: w305 -> [w325 w333]
          frame False {
            n115 = call-dynamic "get_image.vi"("error in (no error)"=w326, "index"=w329, "ImageCollection in"=w325) -> ("error out"=w332:errorcluster, "Image.lvclass"=w331:refnum<class "Image.lvclass">, "ImageCollection out"=w327:T13)  [unwired: 6 in]
            n116 = call-dynamic "get_IMAQ_ref.vi"("error in (no error)"=w332, "Image.lvclass in"=w331) -> ("error out"=w328:errorcluster, "Image"=→"Image":T1)  [unwired: 5 in, 3 out]
          }
          frame True {
          }
        }
      }
      event "Image": Mouse Up {
        n117 = event-data() -> ()  [unwired: 1 in, 1 out]
        n118 = Unbundle By Name(w365) -> ("ROImode"=w367:T10, "current frame index"=w369:i32, "ROI (frames).ROI"=w366:T17)
        n119 = invoke on="Image" class="ImageControl" method="Get Last Event"(error in=w363) -> (error out=w364:errorcluster, "Tool"=w374:i32, "Coordinates"=w371:i32[])  [unwired: 7 in, 5 out]
        n120 = Index Array(array=w371) -> (element #1=w373:i32, element #2=w370:i32)  [unwired: 2 in]
        n121 = Build Array(w373, w370, w369) -> (w372:i32[])
        n122 = To Double Precision Float(number=w372) -> (double precision float=w368:dbl[])
        n123 = case "Which ROI mode?" shown="\"PointCollection\"" w367 {
          tunnel: [w383 w386 w410] -> w355
          tunnel: [w382 w385 w409] -> w353
          tunnel: w374 -> [_ _ w408]
          tunnel: w364 -> [w383 w393 w407]
          tunnel: w369 -> [_ _ w406]
          tunnel: w368 -> [_ _ w405]
          tunnel: w366 -> [_ w395 _]
          tunnel: w365 -> [w382 w394 w404]
          tunnel: w362 -> [w384 w391 w403]
          tunnel: [w384 w390 w402] -> w361
          tunnel: [w381 w388 w401] -> w359
          tunnel: w358 -> [w381 w388 w400]
          tunnel: [_ _ w399] -> w352
          frame "none" {
          }
          frame "IMAQROIs", Default {
            w389 = TRUE ("State Changed?")
            n124 = local read "frame"() -> (w398:i32)
            n125 = property on="Image" class="ImageControl"(error in=w393) -> (error out=w386:errorcluster, "ROI"=w392:T16)  [unwired: 1 in, 1 out]
            n126 = Decrement(x=w398) -> (x-1=w397:i32)
            n127 = Replace Array Subset(array=w395, new element=w392, index=w397) -> (w396:T17)
            n128 = Bundle By Name(cluster=w391, "Data Changed?"=w389, "State Changed?"=w389) -> (w390:T2)
            n129 = Bundle By Name(cluster=w394, "ROI (frames).ROI"=w396, "last action"=last_action_enum."ROIs changed") -> (w385:T3)
          }
          frame "PointCollection" {
            n130 = case "Which tool?" shown="2" w408 {
              tunnel: w407 -> [w414 w439 w478]
              tunnel: [w414 w418 w468] -> w410
              tunnel: w404 -> [w413 w438 w477]
              tunnel: [w413 w440 w467] -> w409
              tunnel: w406 -> [_ _ _]
              tunnel: w405 -> [_ w437 w476]
              tunnel: w403 -> [w412 w421 w473]
              tunnel: [w412 w420 w472] -> w402
              tunnel: [w411 w416 w470] -> w401
              tunnel: w400 -> [w411 w417 w470]
              tunnel: [_ w415 w466] -> w399
              frame Default {
              }
              frame 1 {
                w415 = TRUE  # redraw!
                w419 = TRUE ("State Changed?")
                (unwired) 1 items=["None", "Selection Tool", "Point Tool", "Line Tool", "Rectangle Tool", "Oval Tool", "Polygon Tool", "ClosedFreehandTool", "Annulus Tool", "Rotated Rectangle Tool", "Zoom Tool", "Pan Tool", "Polyline Tool", "Freehand Tool"] ("Tool")
                n131 = call <vilib>:"Intialize Keyboard.vi"("error in (no error)"=w439) -> ("error out"=w435:errorcluster, "device ID"=w434:refnum<k1>)  [unwired: 9 in]
                n132 = call-poly <vilib>:"Acquire Input Data.vi"("device ID"=w434, "error in (no error)"=w435) -> ("device ID"=w433:refnum<k1>, "keys pressed"=w432:T21, "error out"=w436:errorcluster)  [unwired: 15 in]
                n133 = Unbundle By Name(w438) -> ("pointCollection"=w429:refnum<class "PointCollection.lvclass">)
                n134 = call-poly <vilib>:"Close Input Device.vi"("error in (no error)"=w436, "device ID"=w433) -> ("error out"=w422:errorcluster)  [unwired: 8 in]
                n135 = Search 1D Array(1D array=w432, element=T14."DELETE") -> (index of element=w430:i32)  [unwired: 1 in]
                n136 = Greater Or Equal To 0?(x=w430) -> (x >= 0?=w425:bool)
                n137 = call "find_best_match.vi"("radius"=5.0, "error in (no error)"=w422, "location (x/y/z)"=w437, "PointCollection in"=w429) -> ("error out"=w424:errorcluster, "found?"=w426:bool, "point (x/y/z)"=w427:dbl[], "PointCollection out"=w423:refnum<class "PointCollection.lvclass">)  [unwired: 4 in]
                n138 = case "Point found?" shown="True" w426 {
                  tunnel: w427 -> [_ w451]
                  tunnel: [w443 w445] -> w440
                  tunnel: w438 -> [w443 w454]
                  tunnel: w425 -> [_ w453]
                  tunnel: w424 -> [w442 w452]
                  tunnel: [w442 w447] -> w418
                  tunnel: w423 -> [_ w449]
                  tunnel: w417 -> [w441 w444]
                  tunnel: [w441 w444] -> w416
                  frame False {
                  }
                  frame True {
                    n139 = Index Array(array=w451) -> (element=w450:dbl)  [unwired: 1 in]
                    n140 = case "Delete point?" shown="False" w453 {
                      tunnel: [w458 w460] -> w446
                      tunnel: w454 -> [w457 w462]
                      tunnel: w452 -> [w456 w465]
                      tunnel: [w456 w464] -> w447
                      tunnel: w450 -> [w455 w463]
                      tunnel: w449 -> [_ w459]
                      frame False {
                        # "Insert point..."
                        n141 = Bundle By Name(cluster=w457, "selected point ID"=w455) -> (w458:T3)
                      }
                      frame True {
                        n142 = call "delete_point.vi"("error in (no error)"=w465, "point ID"=w463, "PointCollection in"=w459) -> ("error out"=w464:errorcluster, "PointCollection out"=w461:refnum<class "PointCollection.lvclass">)  [unwired: 7 in]
                        n143 = Bundle By Name(cluster=w462, "pointCollection"=w461) -> (w460:T3)
                      }
                    }
                    n144 = Bundle By Name(cluster=w446, "last action"=last_action_enum."ROIs changed") -> (w445:T3)
                  }
                }
                n145 = Bundle By Name(cluster=w421, "Data Changed?"=w419, "State Changed?"=w419) -> (w420:T2)
              }
              frame 2 {
                w466 = TRUE  # redraw!
                w469 = TRUE ("State Changed?")
                (unwired) 2 items=["None", "Selection Tool", "Point Tool", "Line Tool", "Rectangle Tool", "Oval Tool", "Polygon Tool", "ClosedFreehandTool", "Annulus Tool", "Rotated Rectangle Tool", "Zoom Tool", "Pan Tool", "Polyline Tool", "Freehand Tool"] ("Tool")
                n146 = Unbundle By Name(w477) -> ("pointCollection"=w475:refnum<class "PointCollection.lvclass">)
                n147 = call "add_point.vi"("error in (no error)"=w478, "point (x/y/z)"=w476, "PointCollection in"=w475) -> ("error out"=w468:errorcluster, "PointCollection out"=w474:refnum<class "PointCollection.lvclass">)  [unwired: 7 in]
                n148 = Bundle By Name(cluster=w473, "Data Changed?"=w469, "State Changed?"=w469) -> (w472:T2)
                n149 = Bundle By Name(cluster=w477, "last action"=last_action_enum."ROIs changed", "pointCollection"=w474) -> (w467:T3)
              }
            }
          }
        }
        n150 = case "Redraw?" shown="True" w352 {
          tunnel: [w376 w380] -> w356
          tunnel: w355 -> [w376 w379]
          tunnel: [w375 w378] -> w354
          tunnel: w353 -> [w375 w377]
          frame False {
          }
          frame True {
            n151 = call "method_redraw.vi"("Display State In"=w377, "error in (no error)"=w379) -> ("Display State Out"=w378:T3, "error out"=w380:errorcluster)  [unwired: 12 in]
          }
        }
      }
      event Data Change {
        w485 = T16 {"Global Rectangle"=[], "Contours"=[]} ("ROI")
        w489 = TRUE ("State Changed?")
        n152 = event-data() -> ()  [unwired: 1 in, 4 out]
        n153 = property on="Image" class="ImageControl"(error in=w491, "ROI"=w485) -> (error out=w481:errorcluster)  [unwired: 1 in, 1 out]
        n154 = property on="frame" class="Slide (strict)"(error in=w481, "Val(Sgnl)"=1 ("Value (Signaling)")) -> (error out=w487:errorcluster)  [unwired: 1 in, 1 out]
        n155 = call-dynamic "get_number_of_images.vi"("error in (no error)"=w487, "ImageCollection in"=w497) -> ("error out"=w484:errorcluster, "size"=w483:i32, "ImageCollection out"=w496:T13)  [unwired: 7 in]
        n156 = Bundle By Name(cluster=w493, "State Changed?"=w489, "Data Changed?"=w489) -> (w492:T2)
        n157 = Initialize Array(w485, w483) -> (w486:T17)
        n158 = Bundle By Name(cluster=w495, "number of images"=w483, "ROI (frames).ROI"=w486) -> (w494:T3)
        n159 = Greater Than 0?(x=w483) -> (x > 0?=w482:bool)
        n160 = case "Contains at least 1 image?" shown="True" w482 {
          tunnel: w484 -> [w498 w502]
          tunnel: [w498 w499] -> w490
          frame False {
          }
          frame True {
            w501 = T19."Enabled" ("Disabled")
            n161 = property on="button:loadROIs" class="Bool"(error in=w502, "DisabledEnum"=w501) -> (error out=w500:errorcluster)  [unwired: 1 in, 1 out]
            n162 = property on="showHeaderButton" class="Bool"(error in=w500, "DisabledEnum"=w501) -> (error out=w499:errorcluster)  [unwired: 1 in, 1 out]
          }
        }
      }
      event Display State Change {
        n163 = event-data() -> ()  [unwired: 1 in, 1 out]
        n164 = Unbundle By Name(w523) -> ("Refnum"=w522:refnum<vi>)
        n165 = Unbundle By Name(w505) -> ("PlotAreaSize"=w517:cluster{"Width":u32, "Height":u32})
        n166 = Not Equal?(x=cluster{"Width":u32, "Height":u32} {"Width"=0, "Height"=0} ("PlotAreaSize"), y=w517) -> (x != y?=w518:bool)
        n167 = case "new size is NOT zero?" shown="True" w518 {
          tunnel: w522 -> [_ w529]
          tunnel: w517 -> [_ w528]
          tunnel: w521 -> [w525 w527]
          tunnel: [w525 w526] -> w520
          frame False {
          }
          frame True {
            # "write new size"
            n168 = property class="Ctl"(reference=w529, error in=w527, "Container Bounds"=w528) -> (error out=w526:errorcluster)  [unwired: 1 out]
          }
        }
        n169 = Unbundle By Name(w505) -> ("ROI Tool Buttons Visible"=w516:T15, "ROI color"=w510:u32)
        n170 = call <vilib>:"Color to RGB.vi"("Color"=w510) -> ("R"=w512:u8, "G"=w513:u8, "B"=w514:u8)  [unwired: 1 out]
        n171 = Build Array(w512, w513, w514) -> (w515:u8[])
        n172 = Array To Cluster(array=w515) -> (cluster=w511:cluster{"[0]":u8, "[1]":u8, "[2]":u8})
        n173 = property on="Image" class="ImageControl"(error in=w520, "ROI Tool Buttons Visible"=w516, "ROI Color"=w511) -> (error out=w506:errorcluster)  [unwired: 1 in, 1 out]
        n174 = call "method_redraw.vi"("Display State In"=w505, "error in (no error)"=w506) -> ("Display State Out"=w503:T3, "error out"=w504:errorcluster)  [unwired: 12 in]
      }
      event Direction Change {
        # "The direction of the XControl changed from a control to an indicator or vice versa. Update the appearance accordingly."
        n175 = event-data() -> ()  [unwired: 1 in, 4 out]
        n176 = Unbundle By Name(w539) -> ("Indicator?"=w534:bool)
        n177 = Not(x=w534) -> (.not. x?=w535:bool)
        n178 = property on="button:loadImage" class="Bool"(error in=w533, "Visible"=w535) -> (error out=w532:errorcluster)  [unwired: 1 in, 1 out]
      }
      event Panel Resize {
        # "initialize area size"
        n179 = event-data() -> ("OldBnds"=w606:T22, "NewBnds"=w605:T22)  [unwired: 1 in]
        n180 = Unbundle By Name(w559) -> ("Refnum"=w556:refnum<vi>)
        n181 = property class="Ctl"(reference=w556, error in=w558) -> (error out=w557:errorcluster, "Container Bounds"=w553:T23)  [unwired: 1 out]
        n182 = Bundle By Name(cluster=w555, "PlotAreaSize"=w553) -> (w554:T3)
        n183 = Unbundle By Name(w606) -> ("right"=w603:i16, "bottom"=w602:i16)
        n184 = Unbundle By Name(w605) -> ("right"=w604:i16, "bottom"=w601:i16)
        n185 = property on="Image" class="ImageControl"(error in=w557) -> (error out=w600:errorcluster, "Image Area Height"=w596:u32, "Image Area Width"=w599:u32)  [unwired: 1 in, 1 out]
        n186 = Subtract(x=w604, y=w603) -> (x-y=w585:i16)
        n187 = Subtract(x=w601, y=w602) -> (x-y=w595:i16)
        n188 = To Unsigned Long Integer(number=w585) -> (unsigned 32bit integer=w561:u32)
        n189 = Add(x=w561, y=w599) -> (x+y=w598:u32)
        n190 = To Unsigned Long Integer(number=w595) -> (unsigned 32bit integer=w560:u32)
        n191 = Add(x=w560, y=w596) -> (x+y=w597:u32)
        n192 = property on="Image" class="ImageControl"(error in=w600, "Image Area Height"=w597, "Image Area Width"=w598) -> (error out=w594:errorcluster)  [unwired: 1 in, 1 out]
        n193 = To Long Integer(number=w585) -> (32bit integer=w544:i32)
        n194 = Bundle By Name(cluster=w551, "State Changed?"=TRUE ("Data Changed?")) -> (w550:T2)
        n195 = property on="frame" class="Slide (strict)"(error in=w594) -> (error out=w593:errorcluster, "Height"=w592:u32)  [unwired: 1 in, 1 out]
        n196 = Add(x=w560, y=w592) -> (x+y=w591:u32)
        n197 = property on="frame" class="Slide (strict)"(error in=w593, "Height"=w591) -> (error out=w588:errorcluster)  [unwired: 1 in, 1 out]
        n198 = To Long Integer(number=w560) -> (32bit integer=w586:i32)
        n199 = property on="showHeaderButton" class="Bool"(error in=w588) -> (error out=w589:errorcluster, "Top"=w590:i32)  [unwired: 1 in, 1 out]
        n200 = Add(x=w586, y=w590) -> (x+y=w587:i32)
        n201 = property on="showHeaderButton" class="Bool"(error in=w589, "Top"=w587) -> (error out=w562:errorcluster)  [unwired: 1 in, 1 out]
        n202 = property on="progress bar" class="Slide (strict)"(error in=w562) -> (error out=w563:errorcluster, "Width"=w565:u32)  [unwired: 1 in, 1 out]
        n203 = Add(x=w561, y=w565) -> (x+y=w564:u32)
        n204 = property on="progress bar" class="Slide (strict)"(error in=w563, "Width"=w564) -> (error out=w545:errorcluster)  [unwired: 1 in, 1 out]
        n205 = property on="button:loadPoints" class="Bool"(error in=w545) -> (error out=w583:errorcluster, "Left"=w584:i32)  [unwired: 1 in, 1 out]
        n206 = property on="button:savePoints" class="Bool"(error in=w545) -> (error out=w577:errorcluster, "Left"=w580:i32)  [unwired: 1 in, 1 out]
        n207 = property on="button:loadROIs" class="Bool"(error in=w545) -> (error out=w576:errorcluster, "Left"=w579:i32)  [unwired: 1 in, 1 out]
        n208 = property on="button:saveROIs" class="Bool"(error in=w545) -> (error out=w569:errorcluster, "Left"=w570:i32)  [unwired: 1 in, 1 out]
        n209 = property on="button:loadImage" class="Bool"(error in=w545) -> (error out=w567:errorcluster, "Left"=w547:i32)  [unwired: 1 in, 1 out]
        n210 = property on="button:saveLinear" class="Bool"(error in=w545) -> (error out=w541:errorcluster, "Left"=w543:i32)  [unwired: 1 in, 1 out]
        n211 = Add(x=w544, y=w584) -> (x+y=w582:i32)
        n212 = Add(x=w544, y=w580) -> (x+y=w581:i32)
        n213 = Add(x=w544, y=w579) -> (x+y=w578:i32)
        n214 = Add(x=w544, y=w570) -> (x+y=w571:i32)
        n215 = Add(x=w544, y=w547) -> (x+y=w546:i32)
        n216 = Add(x=w544, y=w543) -> (x+y=w542:i32)
        n217 = property on="button:loadPoints" class="Bool"(error in=w583, "Left"=w582) -> (error out=w575:errorcluster)  [unwired: 1 in, 1 out]
        n218 = property on="button:savePoints" class="Bool"(error in=w577, "Left"=w581) -> (error out=w573:errorcluster)  [unwired: 1 in, 1 out]
        n219 = property on="button:loadROIs" class="Bool"(error in=w576, "Left"=w578) -> (error out=w572:errorcluster)  [unwired: 1 in, 1 out]
        n220 = property on="button:saveROIs" class="Bool"(error in=w569, "Left"=w571) -> (error out=w568:errorcluster)  [unwired: 1 in, 1 out]
        n221 = property on="button:loadImage" class="Bool"(error in=w567, "Left"=w546) -> (error out=w566:errorcluster)  [unwired: 1 in, 1 out]
        n222 = property on="button:saveLinear" class="Bool"(error in=w541, "Left"=w542) -> (error out=w540:errorcluster)  [unwired: 1 in, 1 out]
        n223 = Merge Errors(w575, w573, w572, w568, w566, w540) -> (w574:errorcluster)
      }
      event Exec State Change {
        w608 = T19."Disabled and Grayed Out" ("Disabled")
        # "initialize area size"
        # "The VI owning the XControl changed from Edit Mode  to Run Mode or vice versa.\nUpdate the appearance accordingly."
        # "Handle Edit Mode & Run Mode\ncase differently"
        n224 = event-data() -> ()  [unwired: 1 in, 1 out]
        n225 = call-dynamic "destroy.vi"("error in (no error)"=w613, "ImageCollection in"=w614) -> ("error out"=w612:errorcluster)  [unwired: 8 in, 1 out]
        n226 = Unbundle By Name(w640) -> ("Run Mode?"=w635:bool, "Refnum"=w624:refnum<vi>)
        n227 = Not(x=w635) -> (.not. x?=w629:bool)
        n228 = property on="frame" class="Slide (strict)"(error in=w612, "Visible"=w629) -> (error out=w630:errorcluster)  [unwired: 1 in, 1 out]
        n229 = property on="progress bar" class="Slide (strict)"(error in=w630, "Visible"=w629) -> (error out=w628:errorcluster)  [unwired: 1 in, 1 out]
        n230 = property on="Image" class="ImageControl"(error in=w628, "ROI"=T16 {"Global Rectangle"=[], "Contours"=[]}) -> (error out=w623:errorcluster)  [unwired: 1 in, 1 out]
        n231 = property class="Ctl"(reference=w624, error in=w623) -> (error out=w611:errorcluster, "Container Bounds"=w622:T23)  [unwired: 1 out]
        n232 = Bundle By Name(cluster=T3 {"current frame index"=0, "number of images"=0, "ROI (frames)"={"ROI"=[]}, "control refs"={"frame"=refnum, "image"=refnum, "saveROIsButton"=refnum, "loadImageSwitch"=refnum, "loadROIsSwitch"=refnum, "saveROIsSwitch"=refnum, "loadImagePath"=refnum, "loadROIPath"=refnum, "redraw"=refnum}, "calibration"={"x"=0.0, "y"=0.0, "x unit"=enum."um", "y unit"=enum."um"}, "xpaths"={"x offset"="", "y offset"="", "z offset"=""}, "offset"=refnum, "XML description"="", "number of ROIs"=0.0, "ROI Tool Buttons Visible"={"Zoom Tool"=FALSE, "Selection Tool"=FALSE, "Pan Tool"=FALSE, "Point Tool"=FALSE, "Line Tool"=FALSE, "Rectangle Tool"=FALSE, "Rotated Rectangle Tool"=FALSE, "Polyline Tool"=FALSE, "Polygon Tool"=FALSE, "Freehand Tool"=FALSE, "Closed Freehand Tool"=FALSE, "Ellipse Tool"=FALSE, "Annulus Tool"=FALSE}, "ROI color"=0, "enable ROI numbering?"=FALSE, "selected path to save ROIs"=path "", "starting path"=path "", "loaded image path"=path "", "array of overlays"=[], "pointCollection"=refnum, "ROImode"=enum."none", "selected point ID"=0.0, "point radius"=0, "point colours"=[], "PlotAreaSize"={"Width"=0, "Height"=0}, "last action"=enum."not specified"} ("State"), "control refs"=w618, "ROI Tool Buttons Visible"=T15 {"Zoom Tool"=TRUE, "Selection Tool"=TRUE, "Pan Tool"=TRUE, "Point Tool"=TRUE, "Line Tool"=TRUE, "Rectangle Tool"=TRUE, "Rotated Rectangle Tool"=TRUE, "Polyline Tool"=TRUE, "Polygon Tool"=TRUE, "Freehand Tool"=TRUE, "Closed Freehand Tool"=TRUE, "Ellipse Tool"=TRUE, "Annulus Tool"=FALSE}, "point radius"=5, "PlotAreaSize"=w622) -> (w639:T3)
        n233 = property on="button:loadROIs" class="Bool"(error in=w611, "DisabledEnum"=w608) -> (error out=w632:errorcluster)  [unwired: 1 in, 1 out]
        n234 = Bundle By Name(cluster=w637, "State Changed?"=TRUE) -> (w636:T2)
        n235 = local write "Image"(T1 refnum ("Image")) -> ()
        n236 = property on="button:saveROIs" class="Bool"(error in=w632, "DisabledEnum"=w608) -> (error out=w627:errorcluster)  [unwired: 1 in, 1 out]
        n237 = property on="showHeaderButton" class="Bool"(error in=w627, "DisabledEnum"=w608) -> (error out=w625:errorcluster)  [unwired: 1 in, 1 out]
        n238 = property on="button:loadPoints" class="Bool"(error in=w625, "DisabledEnum"=w608) -> (error out=w626:errorcluster)  [unwired: 1 in, 1 out]
        n239 = property on="button:savePoints" class="Bool"(error in=w626, "DisabledEnum"=w608) -> (error out=w610:errorcluster)  [unwired: 1 in, 1 out]
        n240 = property on="button:saveLinear" class="Bool"(error in=w610, "DisabledEnum"=w608) -> (error out=w609:errorcluster)  [unwired: 1 in, 1 out]
        "progress bar" <- u8 0 ("progress bar")
      }
    }
    "event case no." <- w25
    n241 = Wait (ms)(milliseconds to wait=u32 0) -> ()  [unwired: 1 out]
    n242 = call "conditional_error_clearer.vi"("error in (no error)"=w30, "array of clearable error codes"=w29) -> ("error out"=w31:errorcluster)  [unwired: 9 in]
    n243 = Unbundle By Name(w31) -> ("status"=w33:bool)
    n244 = Or(x=w33, y=w35) -> (x .or. y?=w34:bool)
  }
  "Display State Out" <- w19
  "Data Out" <- w22
  "Action" <- w18
  n245 = call <vilib>:"Simple Error Handler.vi"("error in (no error)"=w15) -> ("error out"=→"error out":errorcluster)  [unwired: 4 in, 4 out]
